vi "Reset Board Appearance.vi"(8 "error in (no error)":errorcluster, 11 "Grid Screen in":refnum<class "Grid Screen.lvclass">) -> (0 "error out":errorcluster, 3 "Grid Screen out":refnum<class "Grid Screen.lvclass">)   [LabVIEW 2024, in "Grid Screen.lvlib" / "Grid Screen.lvclass"]
uses:
  Grid Screen.lvclass
  Grid Screen.lvclass/Grid Screen.ctl
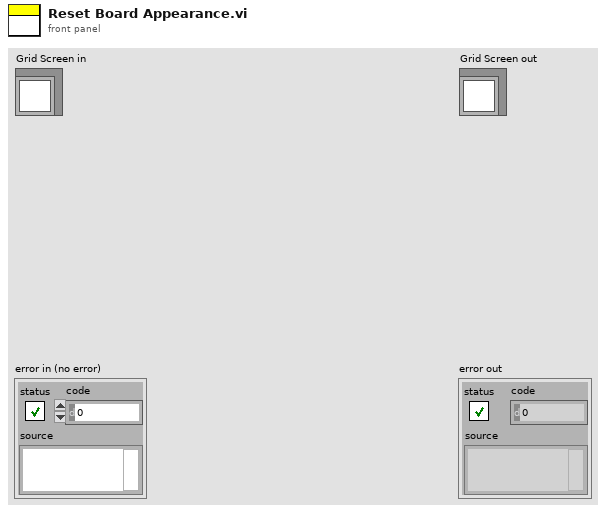
[diagram p1: front panel]
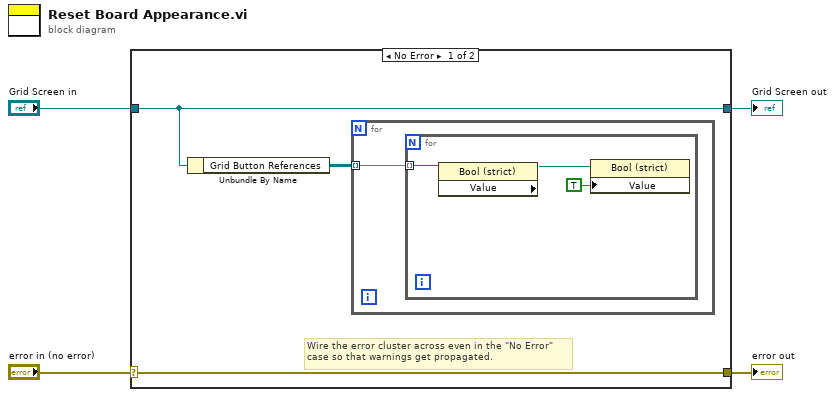
[diagram p0: block diagram]
diagram:
  n1 = case shown="No Error" "error in (no error)" {
    selector: "error in (no error)" -> [w7 w13]
    tunnel: [w7 w13] -> w3
    tunnel: [w6 w12] -> w1
    tunnel: "Grid Screen in" -> [w6 w12]
    frame No Error {
      # "Wire the error cluster across even in the \"No Error\"\ncase so that warnings get propagated."
      n2 = Unbundle By Name(w6) -> ("Grid Button References"=w5:refnum<vi>[][])
      n3 = for {
        tunnel: w5 -> [w8] mode=indexing
        n4 = for {
          tunnel: w8 -> [w11] mode=indexing
          n5 = property class="Bool (strict)" props=["Value"](reference=w11) -> (reference out=w10:refnum<vi>)  [unwired: 1 in, 2 out]
          n6 = property class="Bool (strict)"(reference=w10, "Value"=TRUE) -> ()  [unwired: 1 in, 2 out]
        }
      }
    }
    frame Error {
    }
  }
  "error out" <- w3
  "Grid Screen out" <- w1
